vi "UpdateUserInterface.vi"(8 "error in (no error)":errorcluster, 10 "DataExchange":T2, 11 "QPDController in":refnum<class "QPDController.lvclass">) -> (0 "error out":errorcluster, 2 "DataExchange Out":T2, 3 "QPDController out":refnum<class "QPDController.lvclass">)   [LabVIEW 2020, in "QPDController.lvlib" / "QPDController.lvclass"]
uses:
  QPDController.lvclass
  Model/Hardware Abstraction Layer/Component/Device/Device/DataExchange.ctl
  QPDController.lvclass/QPDController.ctl
  Model/Hardware Abstraction Layer/Component/GenericActor/GenericActor/GenericController.lvclass
  Interface/DataListener/DataListener.lvclass
panel:
  in  "Cluster":T1 {"QPD  Sum" format="%#_13g"; "QPD Voltage Y" format="%#_13g"; "QPD Voltage X" format="%#_13g"}
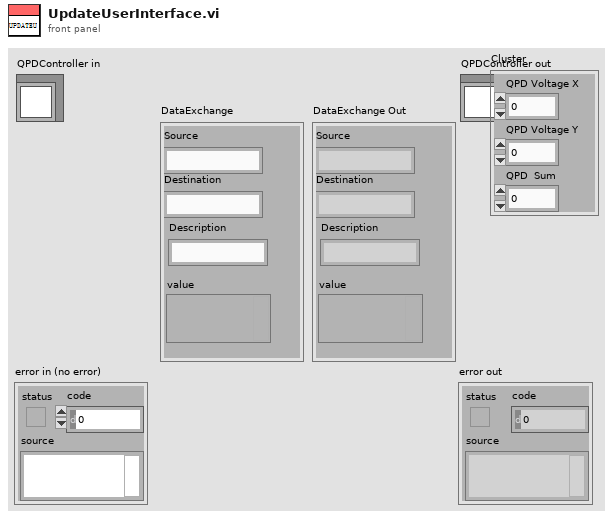
[diagram p1: front panel]
types:
  T1 = cluster{"QPD Voltage X":dbl, "QPD Voltage Y":dbl, "QPD  Sum":dbl}
  T2 = typedef "DataListener.lvclass/DataExchange.ctl" = cluster{"Source":string, "Destination":string, "Description":string, "value":variant}
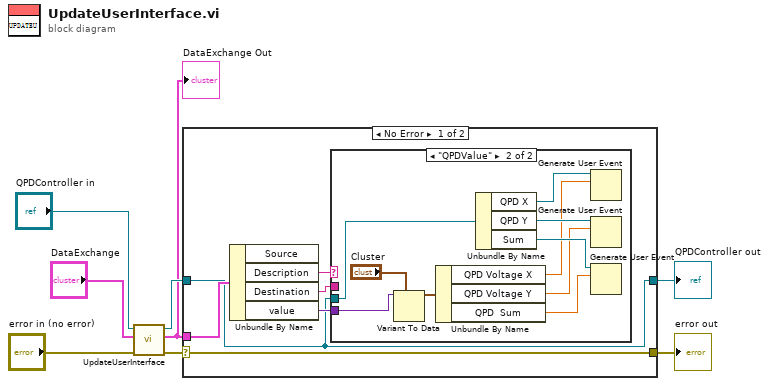
[diagram p0: block diagram]
diagram:
  n1 = call-parent "UpdateUserInterface.vi"("error in (no error)"="error in (no error)", "DataExchange"="DataExchange", "GenericController in"="QPDController in") -> ("error out"=w4:errorcluster, "DataExchange Out"=w1:T2, "GenericController out"=w5:refnum<class "QPDController.lvclass">)  [unwired: 6 in]
  "DataExchange Out" <- w1
  n2 = case shown="No Error" w4 {
    selector: w4 -> [w14 w26]
    tunnel: [w14 w26] -> w2
    tunnel: [w9 w25] -> w3
    tunnel: w5 -> [w9 w25]
    tunnel: w1 -> [w13 _]
    frame No Error {
      n3 = Unbundle By Name(w13) -> ("Description"=w10:string, "Destination"=w11:string, "value"=w12:variant)  [unwired: 1 out]
      n4 = case shown="\"QPDValue\"" w10 {
        tunnel: w12 -> [_ w24]
        tunnel: w11 -> [_ _]
        tunnel: w9 -> [_ w23]
        frame "False", Default {
        }
        frame "QPDValue" {
          n5 = Variant To Data(type="Cluster", Variant=w24) -> (data=w19:T1)  [unwired: 1 in, 1 out]
          n6 = Unbundle By Name(w19) -> ("QPD Voltage X"=w18:dbl, "QPD Voltage Y"=w17:dbl, "QPD  Sum"=w16:dbl)
          n7 = Unbundle By Name(w23) -> ("QPD X"=w22:refnum<user-event>, "QPD Y"=w21:refnum<user-event>, "Sum"=w20:refnum<user-event>)
          n8 = Generate User Event(user event=w22, event data cluster=w18) -> ()  [unwired: 2 in, 2 out]
          n9 = Generate User Event(user event=w21, event data cluster=w17) -> ()  [unwired: 2 in, 2 out]
          n10 = Generate User Event(user event=w20, event data cluster=w16) -> ()  [unwired: 2 in, 2 out]
        }
      }
    }
    frame Error {
    }
  }
  "error out" <- w2
  "QPDController out" <- w3
